vi "Timer2.vi"(8 "error out":errorcluster) -> (0 "errout":errorcluster caption="sortie d'erreur", 4 "30s?":bool)   [LabVIEW 2020]
uses:
  OP500/VG/VG_progressBar.vi
panel:
  out "Glissière":dbl(slide) scale=0.0..30.0
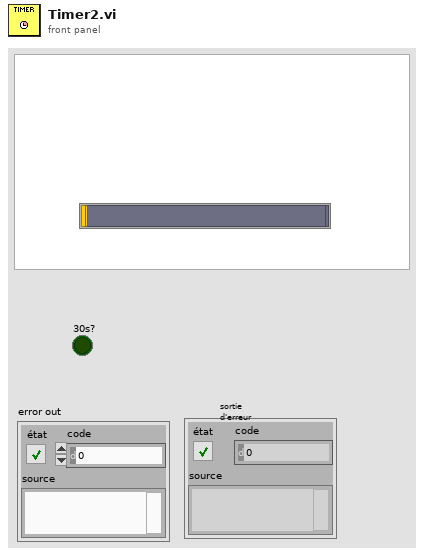
[diagram p1: front panel]
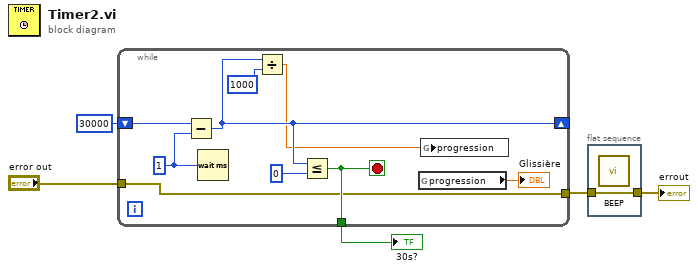
[diagram p0: block diagram]
diagram:
  n1 = while {
    shift-right: [w10] -> _
    shift-left: u32 30000 ("attente (ms)") -> [w14]
    tunnel: [w9] -> w3
    tunnel: "error out" -> [w7]
    tunnel: [w7] -> w2
    stop <- w9 stop-if-true
    w12 = u32 1 ("attente (ms)")
    n2 = Subtract(x=w14, y=w12) -> (x-y=w10:u32)
    n3 = Wait (ms)(milliseconds to wait=w12) -> ()  [unwired: 1 out]
    n4 = Divide(x=w10, y=u32 1000) -> (x/y=w8:dbl)
    n5 = Less Or Equal?(x=w10, y=u32 0) -> (x <= y?=w9:bool)
    n6 = global read "VG_progressBar.vi" "progression"() -> (→"Glissière":dbl)
    n7 = global write "VG_progressBar.vi" "progression"(w8) -> ()
  }
  "30s?" <- w3
  n8 = flat-sequence {
    tunnel: [w15] -> w1
    tunnel: w2 -> [w15]
    frame #0 {
      n9 = call "BEEP.vi"() -> ()  [unwired: 12 in]
    }
  }
  "errout" <- w1
